vi "ABCFirstKickerRole.vi"(7 "first call":bool, 8 "error in (no error) 2":errorcluster, 9 "Game in":refnum<class "Game.lvclass">, 10 "Tactic index in":i32, 11 "ABCFirstKickerRole in":refnum<class "ABCFirstKickerRole.lvclass">) -> (0 "error out 2":errorcluster, 1 "tactic index":i32, 2 "Robot out":refnum<class "Robot.lvclass">, 3 "ABCFirstKickerRole out":refnum<class "ABCFirstKickerRole.lvclass">)   [LabVIEW 2023, in "ABCFirstKickerRole.lvclass"]
uses:
  ABCFirstKickerRole.lvclass
  C:/Users/lucio/Desktop/roboime/SSL_AI/Role_class/Role.lvclass
  Game_class/Game.lvclass
  Robot_class/Robot.lvclass
  Role_class/Role.lvclass/Role.ctl
  Tacticbook_class/Tacticbook.lvclass/Tacticbook.ctl
  FollowAttackerTactic_class/FollowAttackerTactic.lvclass/FollowAttackerTactic.ctl
  KickToPassReceiverTactic_class/KickToPassReceiverTacticStates.ctl
  KickToPassReceiverTactic_class/KickToPassReceiverTactic.lvclass/KickToPassReceiverTactic.ctl
  Tacticbook_class/Read FollowAttackerTactic.vi
  FollowAttackerTactic_class/Read States.vi
  Tacticbook_class/Write FollowAttackerTactic.vi
  KickToPassReceiverTactic_class/Read States.vi
  Role_class/Read Tacticbook.vi
  Role_class/Write Tacticbook.vi
  Role_class/Write tactic_index.vi
  Role_class/Read RobotRef.vi
  Tacticbook_class/Tacticbook.lvclass
  FollowAttackerTactic_class/FollowAttackerTactic.lvclass
  KickToPassReceiverTactic_class/KickToPassReceiverTactic.lvclass
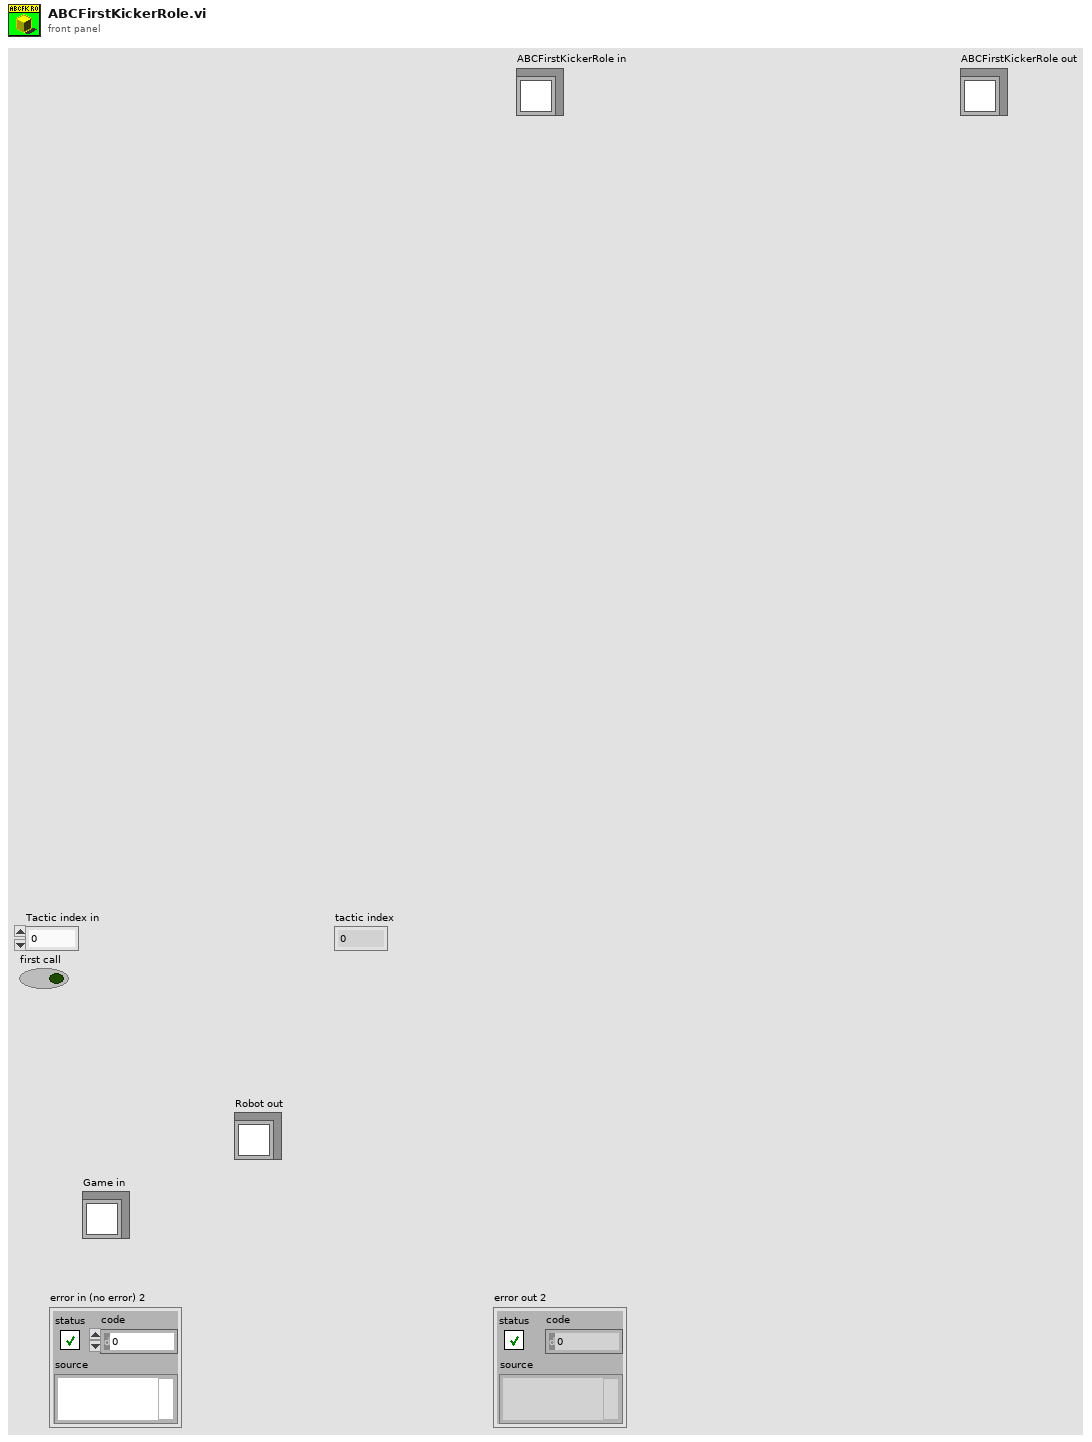
[diagram p1: front panel]
types:
  T1 = typedef "KickToPassReceiverTacticStates.ctl" = enum16{"Halt", "GoToReceiveTable", "KickToPassReceiver", "WaitPass", "Exit"}
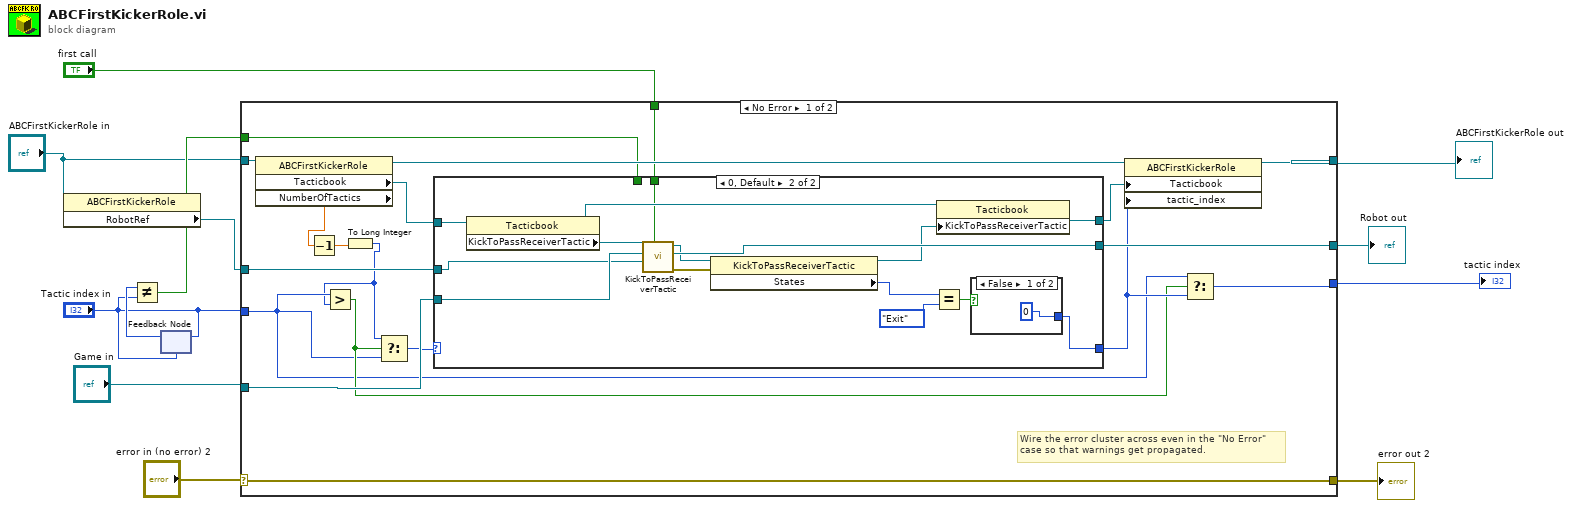
[diagram p0: block diagram]
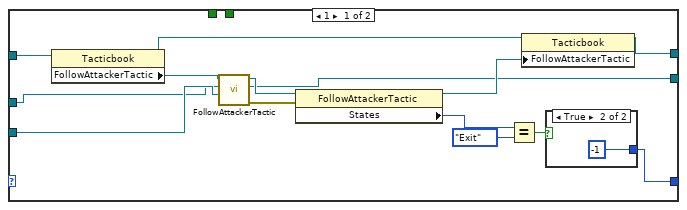
[diagram p2: hidden frame]
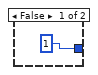
[diagram p3: hidden frame]
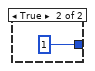
[diagram p4: hidden frame]
diagram:
  n1 = property class="ABCFirstKickerRole"(reference="ABCFirstKickerRole in") -> ("RobotRef"=w10:refnum<class "Robot.lvclass">)  [unwired: 1 in, 2 out]
  n2 = feedback #1("Tactic index in") -> (w6:i32)
  n3 = Not Equal?(x=w6, y="Tactic index in") -> (x != y?=w4:bool)
  n4 = feedback-in #1("Tactic index in") -> ()
  n5 = case shown="No Error" "error in (no error) 2" {
    selector: "error in (no error) 2" -> [w31 w67]
    tunnel: [w31 w67] -> w11
    tunnel: [w29 w66] -> w1
    tunnel: "ABCFirstKickerRole in" -> [w30 w66]
    tunnel: w10 -> [w26 w65]
    tunnel: [w25 w65] -> w3
    tunnel: "Game in" -> [w23 _]
    tunnel: [w21 _] -> w9
    tunnel: "Tactic index in" -> [w18 _]
    tunnel: "first call" -> [w16 _]
    tunnel: w4 -> [w13 _]
    frame No Error {
      # "Wire the error cluster across even in the \"No Error\"\ncase so that warnings get propagated."
      n6 = property class="ABCFirstKickerRole"(reference=w30) -> (reference out=w28:refnum<class "ABCFirstKickerRole.lvclass">, "Tacticbook"=w27:refnum<class "Tacticbook.lvclass">, "NumberOfTactics"=w17:dbl)  [unwired: 1 in, 1 out]
      n7 = Decrement(x=w17) -> (x-1=w15:dbl)
      n8 = To Long Integer(number=w15) -> (32bit integer=w14:i32)
      n9 = Greater?(x=w18, y=w14) -> (0:w19:bool)
      n10 = Select(t=w14, s=w19, f=w18) -> (s? t:f=w20:i32)
      n11 = case shown="0, Default" w20 {
        tunnel: [w39 w50] -> w22
        tunnel: w27 -> [w45 w62]
        tunnel: w26 -> [w36 w53]
        tunnel: [w34 w61] -> w25
        tunnel: [w42 w57] -> w24
        tunnel: w23 -> [w37 w54]
        tunnel: w16 -> [_ w49]
        tunnel: w13 -> [_ _]
        frame 1 {
          n12 = property class="Tacticbook"(reference=w45) -> (reference out=w44:refnum<class "Tacticbook.lvclass">, "FollowAttackerTactic"=w38:refnum<class "FollowAttackerTactic.lvclass">)  [unwired: 1 in, 1 out]
          n13 = call-dynamic "FollowAttackerTactic.vi"("Game in"=w37, "Robot"=w36, "FollowAttackerTactic in"=w38) -> ("error out"=w33:errorcluster, "Robot out"=w34:refnum<class "Robot.lvclass">, "FollowAttackerTactic out"=w35:refnum<class "FollowAttackerTactic.lvclass">)  [unwired: 6 in]
          n14 = property class="FollowAttackerTactic"(reference=w35, error in=w33) -> (reference out=w43:refnum<class "FollowAttackerTactic.lvclass">, "States"=w40:enum16{"Exit", "FollowAttacker"})  [unwired: 1 out]
          n15 = Equal?(x=w40, y=enum16{"Exit", "FollowAttacker"}."Exit") -> (x = y?=w41:bool)
          n16 = property class="Tacticbook"(reference=w44, "FollowAttackerTactic"=w43) -> (reference out=w42:refnum<class "Tacticbook.lvclass">)  [unwired: 1 in, 1 out]
          n17 = case shown="True" w41 {
            tunnel: [1 -1] -> w39
            frame False {
            }
            frame True {
            }
          }
        }
        frame 0, Default {
          n18 = property class="Tacticbook"(reference=w62) -> (reference out=w59:refnum<class "Tacticbook.lvclass">, "KickToPassReceiverTactic"=w56:refnum<class "KickToPassReceiverTactic.lvclass">)  [unwired: 1 in, 1 out]
          n19 = call "KickToPassReceiverTactic.vi"("first call"=w49, "Robot"=w53, "Game in"=w54, "KickToPassReceiverTactic in"=w56) -> ("error out"=w60:errorcluster, "Robot out"=w61:refnum<class "Robot.lvclass">, "KickToPassReceiverTactic out"=w55:refnum<class "KickToPassReceiverTactic.lvclass">)  [unwired: 5 in]
          n20 = property class="KickToPassReceiverTactic"(reference=w55, error in=w60) -> (reference out=w58:refnum<class "KickToPassReceiverTactic.lvclass">, "States"=w51:T1)  [unwired: 1 out]
          n21 = Equal?(x=w51, y=KickToPassReceiverTacticStates."Exit") -> (x = y?=w52:bool)
          n22 = property class="Tacticbook"(reference=w59, "KickToPassReceiverTactic"=w58) -> (reference out=w57:refnum<class "Tacticbook.lvclass">)  [unwired: 1 in, 1 out]
          n23 = case shown="False" w52 {
            tunnel: [0 1] -> w50
            frame False {
            }
            frame True {
            }
          }
        }
      }
      n24 = property class="ABCFirstKickerRole"(reference=w28, "Tacticbook"=w24, "tactic_index"=w22) -> (reference out=w29:refnum<class "ABCFirstKickerRole.lvclass">)  [unwired: 1 in, 1 out]
      n25 = Select(t=w18, s=w19, f=w22) -> (s? t:f=w21:i32)
    }
    frame Error {
    }
  }
  "ABCFirstKickerRole out" <- w1
  "error out 2" <- w11
  "tactic index" <- w9
  "Robot out" <- w3
